vi "F Dwf Analog In Channel Range Steps.vi"(8 "error in (no error)":errorcluster, 9 "pnSteps":i32, 10 "rgVoltsStep":dbl[](array[numeric])=[0.0, 0.0, 0.0, 0.0, 0.0, 0.0, 0.0, 0.0, 0.0, 0.0, 0.0, 0.0, 0.0, 0.0, 0.0, 0.0, 0.0, 0.0, 0.0, 0.0, 0.0, 0.0, 0.0, 0.0, 0.0, 0.0, 0.0, 0.0, 0.0, 0.0, 0.0, 0.0], 11 "hdwf":i32) -> (0 "error out":errorcluster, 1 "pnSteps out":i32, 2 "rgVoltsStep out":dbl[](array[numeric]), 3 "function return":i32)   [LabVIEW 2021, in "Olasdwf.lvlib"]
doc: "DWFAPI int FDwfAnalogInChannelRangeSteps(HDWF hdwf, double rgVoltsStep[32], int *pnSteps);"
uses:
  Olasdwf.lvlib
  Windows/System32/dwf.dll
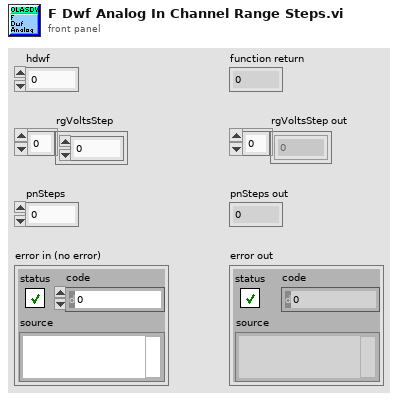
[diagram p1: front panel]
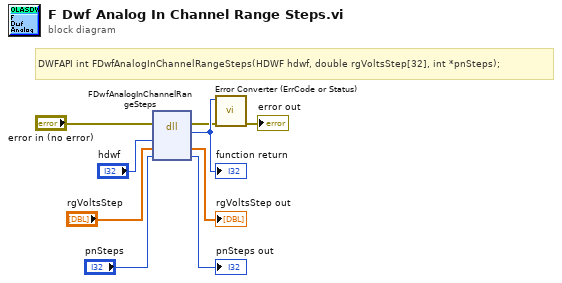
[diagram p0: block diagram]
diagram:
  # "DWFAPI int FDwfAnalogInChannelRangeSteps(HDWF hdwf, double rgVoltsStep[32], int *pnSteps);"
  n1 = dll-call lib="/Windows/System32/dwf.*" fn="FDwfAnalogInChannelRangeSteps"(error in="error in (no error)", "hdwf"="hdwf", "rgVoltsStep"="rgVoltsStep", "pnSteps"="pnSteps") -> (error out=w2:errorcluster, w9:i32, "rgVoltsStep"=→"rgVoltsStep out":dbl[], "pnSteps"=→"pnSteps out":i32)  [unwired: 3 in, 1 out]
  "function return" <- w9
  n2 = call "Error Converter (ErrCode or Status).vi"("error in (no error)"=w2, "error code"=w9) -> ("error out"=→"error out":errorcluster)  [unwired: 9 in]
